vi "display_for_michelle.vi"() -> ()   [LabVIEW 2019]
uses:
  <vilib>/Utility/file.llb/Write Delimited Spreadsheet (DBL).vi
  <vilib>/Analysis/Matrix/Datatypes/RealMatrix.ctl
  <vilib>/Analysis/Matrix/NI_Matrix.lvlib
panel:
  out "Timeout":bool
  out "Num trials":u32=204
  out "ISI Time":dbl
  out "Stim TS":dbl
  out "Output":dbl[][](array[numeric])
  out "Output frame":T1
  out "Array temp1":T1
  out "Elapsed Time":dbl
  out "Display":bool=TRUE
  out "Trial":u32=1
  out "reward":dbl[](array[numeric])
  out "stim_id":dbl[](array[numeric])
  out "stim_loaded":dbl
  out "Timings":dbl[](array[numeric])
  out "Stimuli Loaded?":bool
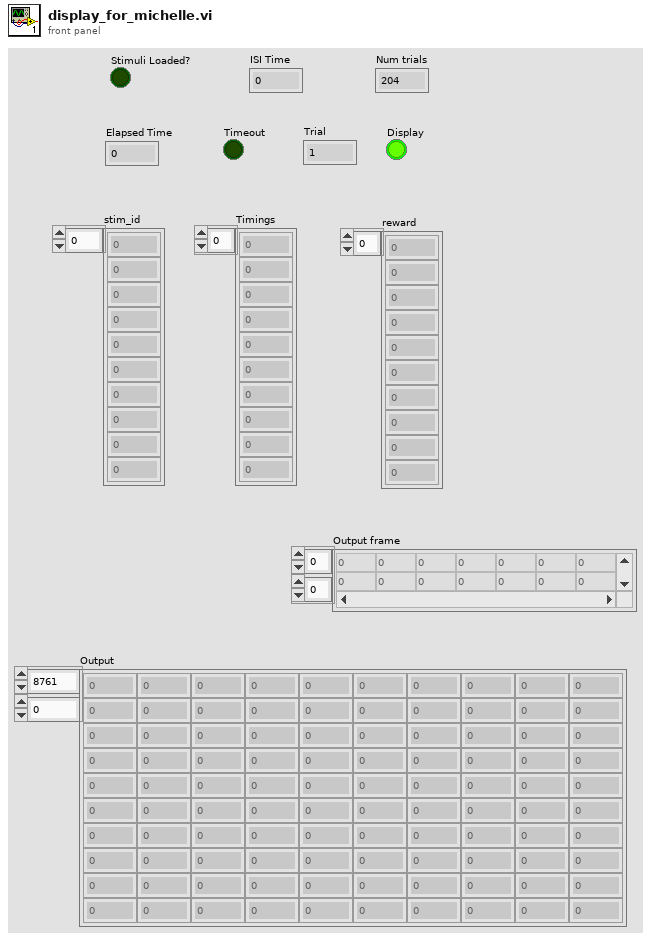
[diagram p1: front panel]
types:
  T1 = typedef "NI_Matrix.lvlib/RealMatrix.ctl" = dbl[][]
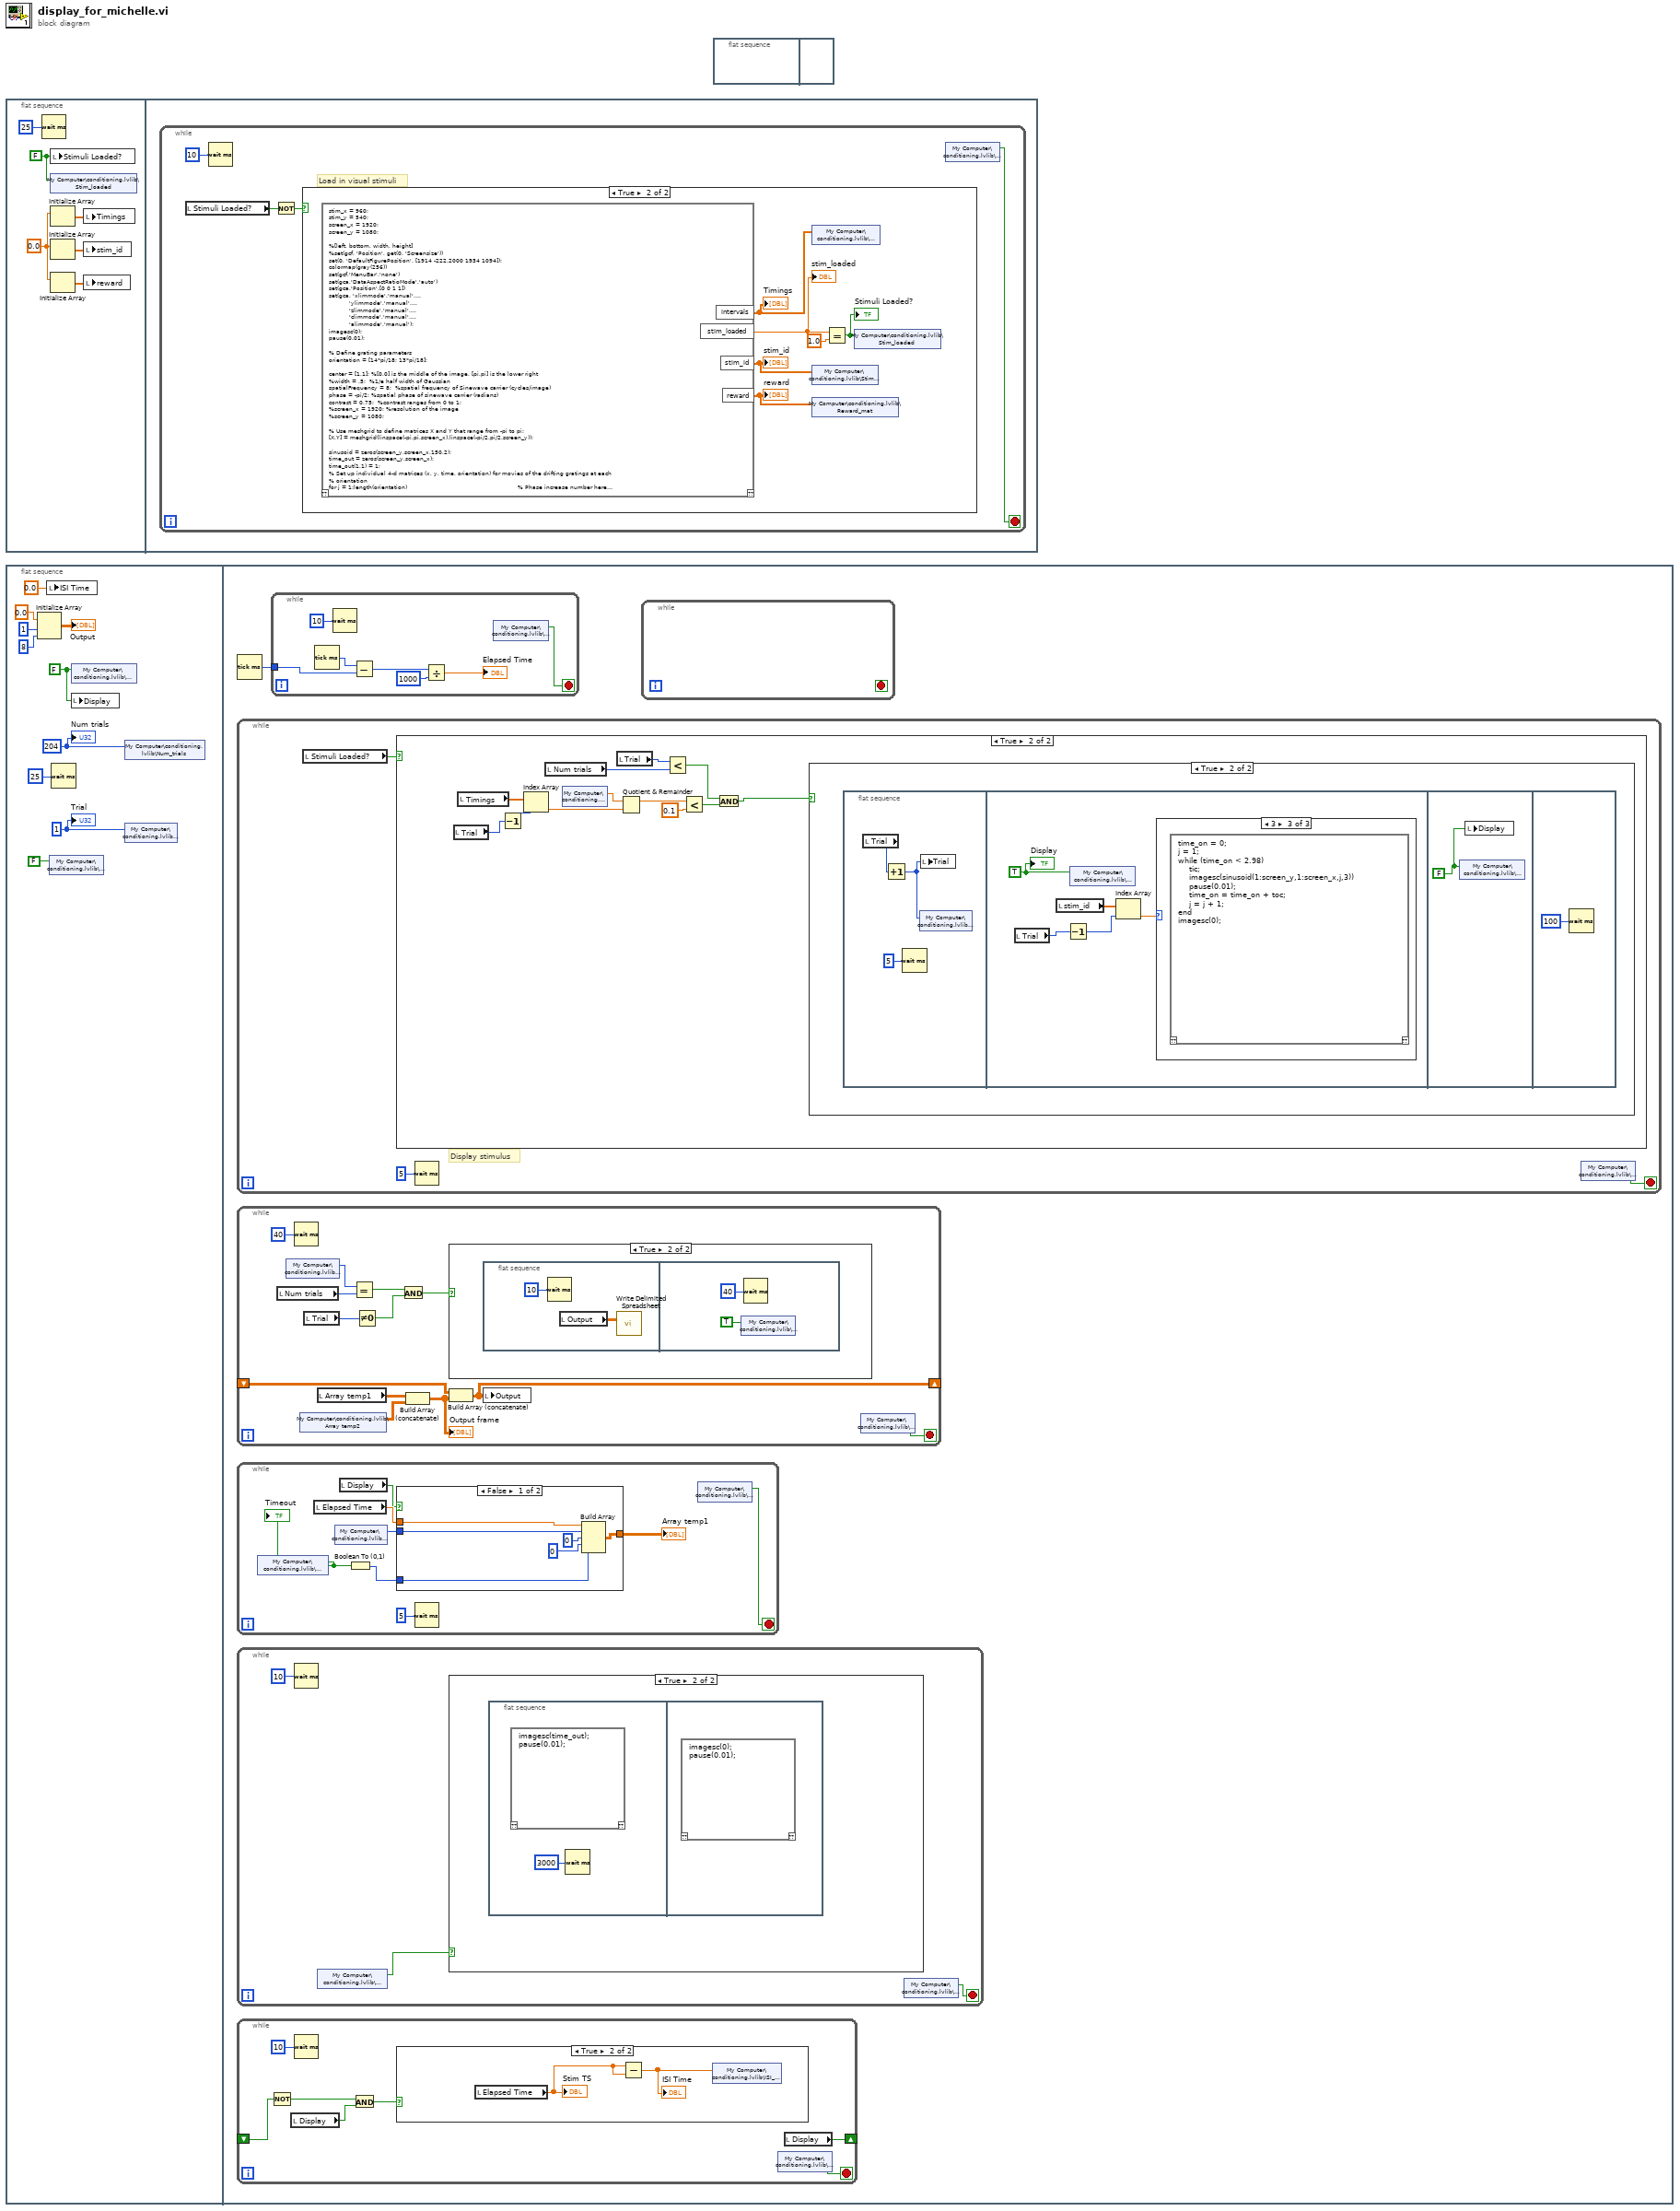
[diagram p0: block diagram]
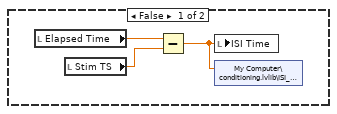
[diagram p4: hidden frame]
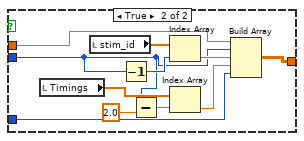
[diagram p5: hidden frame]
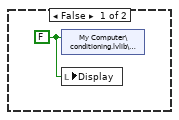
[diagram p8: hidden frame]
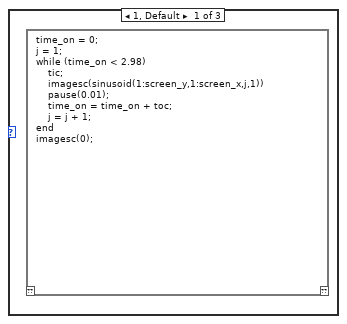
[diagram p9: hidden frame]
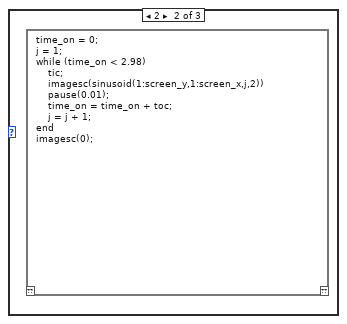
[diagram p10: hidden frame]
diagram:
  n1 = flat-sequence {
    frame #0 {
      w3 = 0.0 ("element")
      w1 = FALSE ("Stimuli Loaded?")
      n2 = Wait (ms)(milliseconds to wait=u32 25) -> ()  [unwired: 1 out]
      n3 = local write "Stimuli Loaded?"(w1) -> ()
      n4 = shared-variable "My Computer\\conditioning.lvlib\\Stim_loaded"(w1) -> ()  [unwired: 1 in, 1 out]
      n5 = Initialize Array(w3) -> (w5:dbl[])  [unwired: 1 in]
      n6 = Initialize Array(w3) -> (w4:dbl[])  [unwired: 1 in]
      n7 = Initialize Array(w3) -> (w2:dbl[])  [unwired: 1 in]
      n8 = local write "Timings"(w5) -> ()
      n9 = local write "stim_id"(w4) -> ()
      n10 = local write "reward"(w2) -> ()
    }
    frame #1 {
      n11 = while {
        stop <- w9 stop-if-true
        # "Load in visual stimuli"
        n12 = local read "Stimuli Loaded?"() -> (w8:bool)
        n13 = Wait (ms)(milliseconds to wait=u32 10) -> ()  [unwired: 1 out]
        n14 = Not(x=w8) -> (.not. x?=w7:bool)
        n15 = case shown="True" w7 {
          frame False {
          }
          frame True {
            n16 = script code="stim_x = 960;\nstim_y = 540;\nscreen_x = 1920;\nscreen_y = 1080;\n\n%[left, bottom, width, height]\n%set(gcf, 'Position', get(0, 'Screensize'))\nset(0, 'DefaultFigurePosition', [1914 -222.2000 1934 1094]);\ncolormap(gray(256))\nset(gcf,'MenuBar','none')\nset(gca,'DataAspectRatioMode','auto')\nset(gca,'Position',[0 0 1 1])\nset(gca, 'xlimmode','manual',...\n           'ylimmode','manual',...\n           'zlimmode','manual',...\n           'climmode','manual',...\n           'alimmode','manual');\nimagesc(0);\npause(0.01);\n\n% Define grating parameters\norientation = [14*pi/18; 13*pi/18];\n\ncenter = [1,1]; %[0,0] is the middle of the image, [pi,pi] is the lower right\n%width = .5;  %1/e half width of Gaussian\nspatialFrequency = 8;  %spatial frequency of Sinewave carrier (cycles/image)\nphase = -pi/2; %spatial phase of sinewave carrier (radians)\ncontrast = 0.75;  %contrast ranges from 0 to 1;\n%screen_x = 1920; %resolution of the image  \n%screen_y = 1080;\n\n% Use meshgrid to define matrices X and Y that range from -pi to pi;\n[X,Y] = meshgrid(linspace(-pi,pi,screen_x),linspace(-pi/2,pi/2,screen_y));\n\nsinusoid = zeros(screen_y,screen_x,150,2);\ntime_out = zeros(screen_y,screen_x);\ntime_out(1,1) = 1;\n% Set up individual 4-d matrices (x, y, time, orientation) for movies of the drifting gratings at each\n% orientation\nfor j = 1:length(orientation)                                                            % Phase increase number here\n    ramp(1:screen_y,1:screen_x,j) = cos(orientation(j))*(X-center(1)) + sin(orientation(j))*(Y-center(2));     %  |\n    for i = 1:150 %Sets the number of frames to define gratings for                   V\n       sinusoid(1:screen_y,1:screen_x,i,j) = contrast*sin(spatialFrequency*ramp(1:screen_y,1:screen_x,j)-...\n           (phase+(2*pi*(i-1)*(-30)/360))); %Number before '/360' sets the phase increase\n    end\nend\n\n%intervals = [ones(1,41)*10 ones(1,41)*11 ones(1,41)*12 ones(1,41)*13 ones(1,40)*14];\nintervals = [ones(1,204)*3];\nstim_id = [ones(1,204)*1];\n%reward = [ones(1,87)*1 ones(1,15)*0 ones(1,87)*1 ones(1,15)*0];\nreward = [ones(1,204)*1];\n\nrand_idx1 = randperm(204);\nrand_idx2 = randperm(204);\nintervals = intervals(rand_idx2);\nstim_id = stim_id(rand_idx2);\nreward = reward(rand_idx2);\n\nstim_loaded = 1;" ("Script Node")() -> ("stim_loaded"=w16:dbl, "intervals"=w11:dbl[], "stim_id"=w12:dbl[], "reward"=w14:dbl[])  [unwired: 1 in, 1 out]
            "stim_loaded" <- w16
            "Timings" <- w11
            "stim_id" <- w12
            "reward" <- w14
            n17 = shared-variable "My Computer\\conditioning.lvlib\\Timings"(w11) -> ()  [unwired: 1 in, 1 out]
            n18 = shared-variable "My Computer\\conditioning.lvlib\\Stim_ID"(w12) -> ()  [unwired: 1 in, 1 out]
            n19 = shared-variable "My Computer\\conditioning.lvlib\\Reward_mat"(w14) -> ()  [unwired: 1 in, 1 out]
            n20 = Equal?(x=w16, y=1.0) -> (x = y?=w13:bool)
            "Stimuli Loaded?" <- w13
            n21 = shared-variable "My Computer\\conditioning.lvlib\\Stim_loaded"(w13) -> ()  [unwired: 1 in, 1 out]
          }
        }
        n22 = shared-variable "My Computer\\conditioning.lvlib\\Stop"() -> (w9:bool)  [unwired: 1 in, 1 out]
      }
    }
  }
  n23 = flat-sequence {
    frame #0 {
      w18 = u32 204
      w24 = FALSE ("Display")
      w26 = u32 1 ("Trial")
      n24 = Initialize Array(0.0 ("element"), 1 ("dimension size"), 8 ("dimension size")) -> (→"Output":dbl[][])
      n25 = local write "ISI Time"(0.0 ("ISI Time")) -> ()
      n26 = shared-variable "My Computer\\conditioning.lvlib\\Stop"(FALSE ("Stop")) -> ()  [unwired: 1 in, 1 out]
      n27 = Wait (ms)(milliseconds to wait=u32 25) -> ()  [unwired: 1 out]
      n28 = shared-variable "My Computer\\conditioning.lvlib\\Display"(w24) -> ()  [unwired: 1 in, 1 out]
      n29 = local write "Display"(w24) -> ()
      n30 = shared-variable "My Computer\\conditioning.lvlib\\Num_trials"(w18) -> ()  [unwired: 1 in, 1 out]
      n31 = shared-variable "My Computer\\conditioning.lvlib\\Trial"(w26) -> ()  [unwired: 1 in, 1 out]
      "Trial" <- w26
      "Num trials" <- w18
    }
    frame #1 {
      n32 = Tick Count (ms)() -> (millisecond timer value=w27:u32)
      n33 = while {
        stop <- w94 stop-if-true
        # "Display stimulus"
        n34 = local read "Stimuli Loaded?"() -> (w93:bool)
        n35 = case shown="True" w93 {
          frame False {
          }
          frame True {
            n36 = local read "Trial"() -> (w96:u32)
            n37 = local read "Timings"() -> (w105:dbl[])
            n38 = Decrement(x=w96) -> (x-1=w97:u32)
            n39 = Index Array(array=w105, index=w97) -> (element=w104:dbl)
            n40 = local read "Num trials"() -> (w100:u32)
            n41 = shared-variable "My Computer\\conditioning.lvlib\\ISI"() -> (w99:dbl)  [unwired: 1 in, 1 out]
            n42 = local read "Trial"() -> (w103:u32)
            n43 = Quotient & Remainder(x=w99, y=w104) -> (x-y*floor(x/y)=w107:dbl)  [unwired: 1 out]
            n44 = Less?(x=w103, y=w100) -> (x < y?=w102:bool)
            n45 = Less?(x=w107, y=0.1) -> (x < y?=w101:bool)
            n46 = And(x=w102, y=w101) -> (x .and. y?=w98:bool)
            n47 = case shown="True" w98 {
              frame False {
                w108 = FALSE ("Display")
                n48 = shared-variable "My Computer\\conditioning.lvlib\\Display"(w108) -> ()  [unwired: 1 in, 1 out]
                n49 = local write "Display"(w108) -> ()
              }
              frame True {
                n50 = flat-sequence {
                  frame #0 {
                    n51 = local read "Trial"() -> (w111:u32)
                    n52 = Increment(x=w111) -> (x+1=w110:u32)
                    n53 = Wait (ms)(milliseconds to wait=u32 5) -> ()  [unwired: 1 out]
                    n54 = shared-variable "My Computer\\conditioning.lvlib\\Trial"(w110) -> ()  [unwired: 1 in, 1 out]
                    n55 = local write "Trial"(w110) -> ()
                  }
                  frame #1 {
                    w115 = TRUE ("Boolean")
                    n56 = local read "Trial"() -> (w113:u32)
                    n57 = local read "stim_id"() -> (w116:dbl[])
                    n58 = Decrement(x=w113) -> (x-1=w112:u32)
                    n59 = shared-variable "My Computer\\conditioning.lvlib\\Display"(w115) -> ()  [unwired: 1 in, 1 out]
                    n60 = Index Array(array=w116, index=w112) -> (element=w114:dbl)
                    n61 = case shown="3" w114 {
                      frame 1, Default {
                        n62 = script code="time_on = 0;\nj = 1;\nwhile (time_on < 2.98)\n    tic;\n    imagesc(sinusoid(1:screen_y,1:screen_x,j,1))\n    pause(0.01);\n    time_on = time_on + toc;\n    j = j + 1;\nend\nimagesc(0);"() -> ()  [unwired: 1 in, 1 out]
                      }
                      frame 2 {
                        n63 = script code="time_on = 0;\nj = 1;\nwhile (time_on < 2.98)\n    tic;\n    imagesc(sinusoid(1:screen_y,1:screen_x,j,2))\n    pause(0.01);\n    time_on = time_on + toc;\n    j = j + 1;\nend\nimagesc(0);"() -> ()  [unwired: 1 in, 1 out]
                      }
                      frame 3 {
                        n64 = script code="time_on = 0;\nj = 1;\nwhile (time_on < 2.98)\n    tic;\n    imagesc(sinusoid(1:screen_y,1:screen_x,j,3))\n    pause(0.01);\n    time_on = time_on + toc;\n    j = j + 1;\nend\nimagesc(0);"() -> ()  [unwired: 1 in, 1 out]
                      }
                    }
                    "Display" <- w115
                  }
                  frame #2 {
                    w117 = FALSE ("Display")
                    n65 = shared-variable "My Computer\\conditioning.lvlib\\Display"(w117) -> ()  [unwired: 1 in, 1 out]
                    n66 = local write "Display"(w117) -> ()
                  }
                  frame #3 {
                    n67 = Wait (ms)(milliseconds to wait=u32 100) -> ()  [unwired: 1 out]
                  }
                }
              }
            }
          }
        }
        n68 = Wait (ms)(milliseconds to wait=u32 5) -> ()  [unwired: 1 out]
        n69 = shared-variable "My Computer\\conditioning.lvlib\\Stop"() -> (w94:bool)  [unwired: 1 in, 1 out]
      }
      n70 = while {
        shift-right: [w85] -> _
        shift-left: _ -> [w86]
        stop <- w88 stop-if-true
        n71 = local read "Num trials"() -> (w80:u32)
        n72 = shared-variable "My Computer\\conditioning.lvlib\\Trial"() -> (w81:u32)  [unwired: 1 in, 1 out]
        n73 = Wait (ms)(milliseconds to wait=u32 40) -> ()  [unwired: 1 out]
        n74 = shared-variable "My Computer\\conditioning.lvlib\\Array temp2"() -> (w83:dbl[][])  [unwired: 1 in, 1 out]
        n75 = local read "Trial"() -> (w78:u32)
        n76 = local read "Array temp1"() -> (w84:T1)
        n77 = Equal?(x=w81, y=w80) -> (x = y?=w79:bool)
        n78 = Not Equal To 0?(x=w78) -> (x != 0?=w77:bool)
        n79 = And(x=w79, y=w77) -> (x .and. y?=w76:bool)
        n80 = Build Array (concatenate)(w84, w83) -> (w82:T1)
        "Output frame" <- w82
        n81 = case shown="True" w76 {
          frame False {
          }
          frame True {
            n82 = flat-sequence {
              frame #0 {
                n83 = Wait (ms)(milliseconds to wait=u32 10) -> ()  [unwired: 1 out]
                n84 = local read "Output"() -> (w90:dbl[][])
                n85 = call-poly <vilib>:"Write Delimited Spreadsheet.vi"("2D data"=w90) -> ()  [unwired: 13 in, 2 out]
              }
              frame #1 {
                n86 = shared-variable "My Computer\\conditioning.lvlib\\Stop"(TRUE) -> ()  [unwired: 1 in, 1 out]
                n87 = Wait (ms)(milliseconds to wait=u32 40) -> ()  [unwired: 1 out]
              }
            }
          }
        }
        n88 = Build Array (concatenate) ("Build Matrix")(w86, w82) -> (w85:T1)
        n89 = local write "Output"(w85) -> ()
        n90 = shared-variable "My Computer\\conditioning.lvlib\\Stop"() -> (w88:bool)  [unwired: 1 in, 1 out]
      }
      n91 = while {
        stop <- w46 stop-if-true
        n92 = shared-variable "My Computer\\conditioning.lvlib\\Timeout"() -> (w45:bool)  [unwired: 1 in, 1 out]
        "Timeout" <- w45
        n93 = local read "Elapsed Time"() -> (w50:dbl)
        n94 = shared-variable "My Computer\\conditioning.lvlib\\Trial"() -> (w48:u32)  [unwired: 1 in, 1 out]
        n95 = local read "Display"() -> (w47:bool)
        n96 = Boolean To (0,1)(Boolean=w45) -> (0, 1=w44:i16)
        n97 = case shown="False" w47 {
          tunnel: w48 -> [w56 w59]
          tunnel: w50 -> [w57 w66]
          tunnel: [w55 w67] -> w49
          tunnel: w44 -> [w52 w61]
          frame False {
            n98 = Build Array(w57, w56, u32 0 ("milliseconds to wait"), 0, w52) -> (w55:T1)
          }
          frame True {
            n99 = local read "Timings"() -> (w64:dbl[])
            n100 = local read "stim_id"() -> (w68:dbl[])
            n101 = Decrement(x=w59) -> (x-1=w63:u32)
            n102 = Subtract(x=w59, y=2.0) -> (x-y=w58:dbl)
            n103 = Index Array(array=w68, index=w63) -> (element=w65:dbl)
            n104 = Index Array(array=w64, index=w58) -> (element=w62:dbl)
            n105 = Build Array(w66, w59, w65, w62, w61) -> (w67:T1)
          }
        }
        "Array temp1" <- w49
        n106 = Wait (ms)(milliseconds to wait=u32 5) -> ()  [unwired: 1 out]
        n107 = shared-variable "My Computer\\conditioning.lvlib\\Stop"() -> (w46:bool)  [unwired: 1 in, 1 out]
      }
      n108 = while {
        stop <- w30 stop-if-true
        n109 = Wait (ms)(milliseconds to wait=u32 10) -> ()  [unwired: 1 out]
        n110 = shared-variable "My Computer\\conditioning.lvlib\\Timeout"() -> (w28:bool)  [unwired: 1 in, 1 out]
        n111 = case shown="True" w28 {
          frame False {
          }
          frame True {
            n112 = flat-sequence {
              frame #0 {
                n113 = script code="imagesc(time_out);\npause(0.01);"() -> ()  [unwired: 1 in, 1 out]
                n114 = Wait (ms)(milliseconds to wait=u32 3000) -> ()  [unwired: 1 out]
              }
              frame #1 {
                n115 = script code="imagesc(0);\npause(0.01);"() -> ()  [unwired: 1 in, 1 out]
              }
            }
          }
        }
        n116 = shared-variable "My Computer\\conditioning.lvlib\\Stop"() -> (w30:bool)  [unwired: 1 in, 1 out]
      }
      n117 = while {
        shift-right: [w36] -> _
        shift-left: _ -> [w35]
        stop <- w38 stop-if-true
        n118 = Not(x=w35) -> (.not. x?=w34:bool)
        n119 = local read "Display"() -> (w33:bool)
        n120 = Wait (ms)(milliseconds to wait=u32 10) -> ()  [unwired: 1 out]
        n121 = And(x=w34, y=w33) -> (x .and. y?=w32:bool)
        n122 = case shown="True" w32 {
          frame False {
            n123 = local read "Elapsed Time"() -> (w39:dbl)
            n124 = local read "Stim TS"() -> (w41:dbl)
            n125 = Subtract(x=w39, y=w41) -> (x-y=w40:dbl)
            n126 = local write "ISI Time"(w40) -> ()
            n127 = shared-variable "My Computer\\conditioning.lvlib\\ISI_Time"(w40) -> ()  [unwired: 1 in, 1 out]
          }
          frame True {
            n128 = local read "Elapsed Time"() -> (w42:dbl)
            "Stim TS" <- w42
            n129 = Subtract(x=w42, y=w42) -> (x-y=w43:dbl)
            "ISI Time" <- w43
            n130 = shared-variable "My Computer\\conditioning.lvlib\\ISI_Time"(w43) -> ()  [unwired: 1 in, 1 out]
          }
        }
        n131 = shared-variable "My Computer\\conditioning.lvlib\\Stop"() -> (w38:bool)  [unwired: 1 in, 1 out]
        n132 = local read "Display"() -> (w36:bool)
      }
      n133 = while {
        tunnel: w27 -> [w72]
        stop <- w69 stop-if-true
        n134 = Tick Count (ms)() -> (millisecond timer value=w73:u32)
        n135 = Wait (ms)(milliseconds to wait=u32 10) -> ()  [unwired: 1 out]
        n136 = Subtract(x=w73, y=w72) -> (x-y=w70:u32)
        n137 = Divide(x=w70, y=u32 1000) -> (x/y=→"Elapsed Time":dbl)
        n138 = shared-variable "My Computer\\conditioning.lvlib\\Stop"() -> (w69:bool)  [unwired: 1 in, 1 out]
      }
      n139 = while {
        stop <- _ stop-if-true
      }
    }
  }
  n140 = flat-sequence {
    frame #0 {
    }
    frame #1 {
    }
  }
